vi "Box IDs Differ by 1 Char.vi"(8 "Error In":errorcluster, 11 "1D String Array":string[](array[string])) -> (0 "Error Out":errorcluster, 2 "Box 2":string, 3 "Box 1":string)   [LabVIEW 2019]
doc: "Given a list of strings, search the list for the first box ID that differs from a subsequent box ID by only 1 character and return both box IDs."
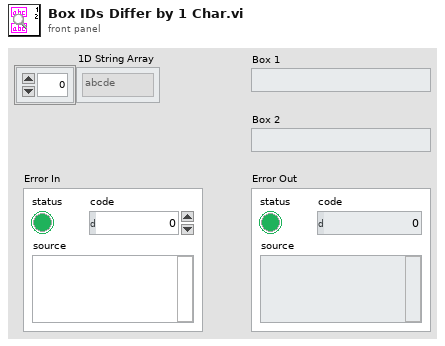
[diagram p1: front panel]
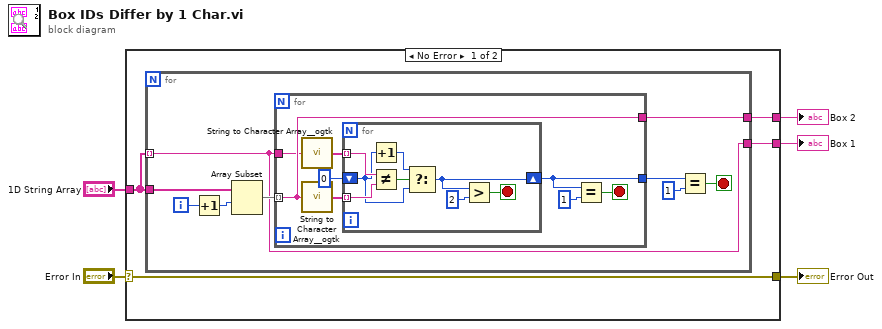
[diagram p0: block diagram]
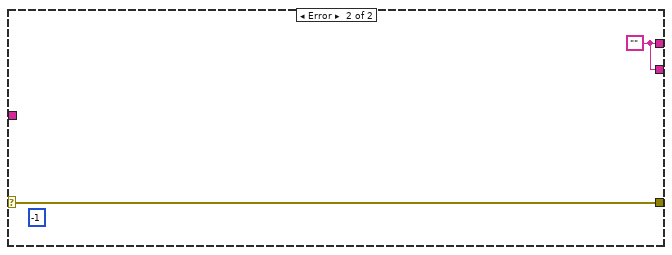
[diagram p2: hidden frame]
diagram:
  n1 = case shown="No Error" "Error In" {
    selector: "Error In" -> [w6 w36]
    tunnel: [w9 w35] -> w5
    tunnel: [w8 w35] -> w4
    tunnel: "1D String Array" -> [w7 _]
    tunnel: [w6 w36] -> w1
    frame No Error {
      n2 = for {
        tunnel: w7 -> [w13] mode=indexing
        tunnel: w7 -> [w16]
        tunnel: [w13] -> w8
        tunnel: [w18] -> w9
        i -> [w17]
        stop <- w10 stop-if-true
        n3 = Increment(x=w17) -> (x+1=w15:i32)
        n4 = Array Subset(array=w16, index=w15) -> (w14:string[])  [unwired: 1 in]
        n5 = for {
          tunnel: [w25] -> w18
          tunnel: w14 -> [w25] mode=indexing
          tunnel: w13 -> [w24]
          tunnel: [w19] -> w11
          stop <- w20 stop-if-true
          n6 = call <userlib>:"String to Character Array__ogtk.vi"("Input String"=w24) -> ("Character Array"=w23:string[])
          n7 = call <userlib>:"String to Character Array__ogtk.vi"("Input String"=w25) -> ("Character Array"=w26:string[])
          n8 = for {
            tunnel: w23 -> [w34] mode=indexing
            tunnel: w26 -> [w33] mode=indexing
            shift-right: [w28] -> w19
            shift-left: 0 -> [w30]
            stop <- w29 stop-if-true
            n9 = Increment(x=w30) -> (x+1=w31:i32)
            n10 = Not Equal?(x=w34, y=w33) -> (x != y?=w32:bool)
            n11 = Select(t=w31, s=w32, f=w30) -> (s? t:f=w28:i32)
            n12 = Greater?(x=w28, y=2) -> (0:w29:bool)
          }
          n13 = Equal?(x=w19, y=1) -> (x = y?=w20:bool)
        }
        n14 = Equal?(x=w11, y=1) -> (x = y?=w10:bool)
      }
    }
    frame Error {
      (unwired) -1
      w35 = ""
    }
  }
  "Box 1" <- w4
  "Box 2" <- w5
  "Error Out" <- w1
